vi "Get ControlRef from ctrlVI.vi"(8 "error in (no error)":errorcluster, 11 "VI ref in":refnum<vi>) -> (0 "error out":errorcluster, 2 "Control ref out":refnum<vi>, 3 "VI ref out":refnum<vi>)   [LabVIEW 2019, in "gRPC Scripting Tools.lvlib"]
uses:
  gRPC Scripting Tools.lvlib
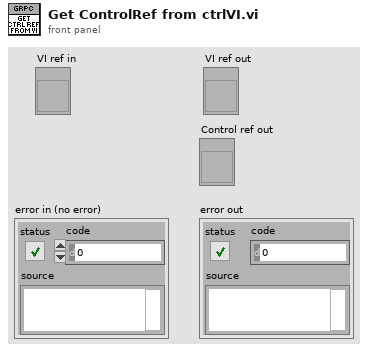
[diagram p1: front panel]
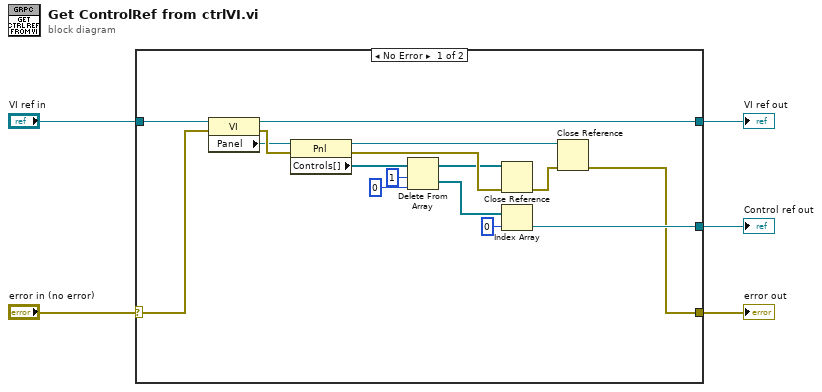
[diagram p0: block diagram]
diagram:
  n1 = case shown="No Error" "error in (no error)" {
    selector: "error in (no error)" -> [w6 w22]
    tunnel: [w17 _] -> w5
    tunnel: "VI ref in" -> [w11 w23]
    tunnel: [w8 w22] -> w3
    tunnel: [w7 w23] -> w2
    frame No Error {
      n2 = property class="VI"(reference=w11, error in=w6) -> (reference out=w7:refnum<vi>, error out=w18:errorcluster, "Panel"=w10:refnum<vi>)
      n3 = property class="Pnl"(reference=w10, error in=w18) -> (reference out=w9:refnum<vi>, error out=w19:errorcluster, "Controls[]"=w12:refnum<vi>[])
      n4 = Delete From Array(array=w12, length=1, index=0) -> (deleted portion=w16:refnum<vi>[], array with subset deleted=w15:refnum<vi>[])
      n5 = Close Reference(reference=w15, error in (no error)=w19) -> (error out=w20:errorcluster)
      n6 = Index Array(array=w16, index=0) -> (element=w17:refnum<vi>)
      n7 = Close Reference(reference=w9, error in (no error)=w20) -> (error out=w8:errorcluster)
    }
    frame Error {
    }
  }
  "error out" <- w3
  "Control ref out" <- w5
  "VI ref out" <- w2
